vi "Write Default Value.vi"(8 "error in":errorcluster, 10 "default value":dbl, 11 "analog channel in":refnum<class "Analog Channel.lvclass">) -> (0 "error out":errorcluster, 3 "analog channel out":refnum<class "Analog Channel.lvclass">)   [LabVIEW 2020, in "Scan Engine Scripting.lvlib" / "Analog Channel.lvclass"]
uses:
  Analog Channel.lvclass
  Analog Channel.lvclass/Analog Channel.ctl
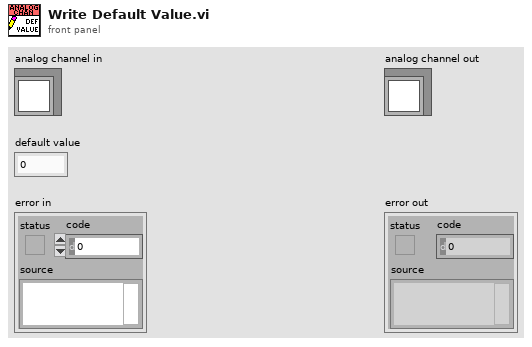
[diagram p1: front panel]
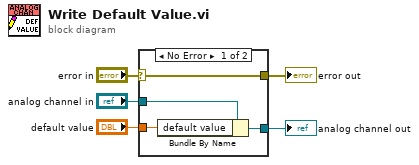
[diagram p0: block diagram]
diagram:
  n1 = case shown="No Error" "error in" {
    selector: "error in" -> [w9 w10]
    tunnel: [w9 w10] -> w4
    tunnel: [w7 w11] -> w2
    tunnel: "analog channel in" -> [w8 w11]
    tunnel: "default value" -> [w6 _]
    frame No Error {
      n2 = Bundle By Name(cluster=w8, "default value"=w6) -> (w7:refnum<class "Analog Channel.lvclass">)
    }
    frame Error {
    }
  }
  "error out" <- w4
  "analog channel out" <- w2
